vi "Handle Error.vi"(8 "error in (no error)":errorcluster caption="错误输入（无错误）", 11 "Log in":refnum<class "Log.lvclass"> caption="操作者输入") -> (0 "error out":errorcluster caption="错误输出", 2 "stop actor?":bool=TRUE caption="停止操作者？", 3 "Log out":refnum<class "Log.lvclass"> caption="操作者输出")   [LabVIEW 2019, in "Log.lvlib" / "Log.lvclass"]
doc: "(<B>Filename</B>: Actor Framework.lvlib:Actor.lvclass:Handle Error.vi)\n\nDefines how the actor handles an error that occurred while processing a message.默认情况下，该方法不执行任何操作，仅停止操作者。"
uses:
  Log.lvclass
  Log.lvclass/Log.ctl
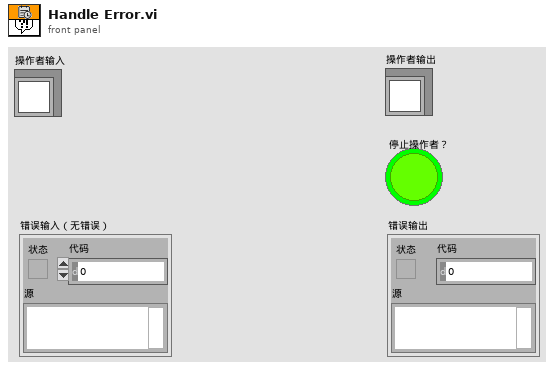
[diagram p1: front panel]
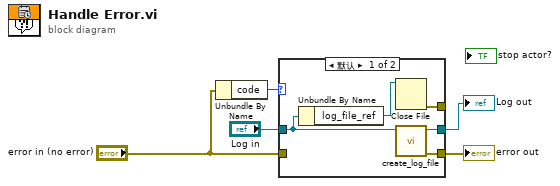
[diagram p0: block diagram]
diagram:
  n1 = Unbundle By Name("error in (no error)") -> ("code"=w5:i32)
  n2 = case shown="默认" w5 {
    tunnel: [w9 _] -> _
    tunnel: "Log in" -> [w8 w12]
    tunnel: [w6 w11] -> w3
    tunnel: [w7 w12] -> w2
    tunnel: "error in (no error)" -> [_ w11]
    frame Default {
      n3 = Unbundle By Name(w8) -> ("log_file_ref"=w10:refnum<file>)
      n4 = Close File(refnum=w10) -> (error out=w9:errorcluster)  [unwired: 1 in, 1 out]
      n5 = call "create_log_file.vi"("Log 输入"=w8) -> ("error out"=w6:errorcluster, "Log 输出"=w7:refnum<class "Log.lvclass">)  [unwired: 9 in]
    }
    frame 43 {
    }
  }
  "Log out" <- w2
  "error out" <- w3
